vi "CalSet_Control.vi"(8 "error in (no error)":errorcluster, 9 "CalSet Control":enum16{"Save", "Delete", "Load"}(ring), 10 "CalSet Filename (*.cal)":string, 11 "NetA_AgNA in":refnum<class "NetA_AgNA.lvclass">) -> (0 "error out":errorcluster, 3 "NetA_AgNA out":refnum<class "NetA_AgNA.lvclass">)   [LabVIEW 2014, in "NetA_AgNA.lvclass"]
doc: "This allows user to load, save, or delete CalSet files. These files are non-proprietary and stored outside of the Keysight folders."
uses:
  NetA_AgNA.lvclass
  NetA_AgNA.lvclass/NetA_AgNA.ctl
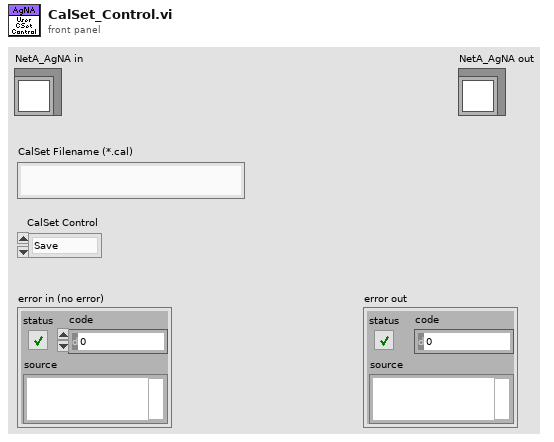
[diagram p1: front panel]
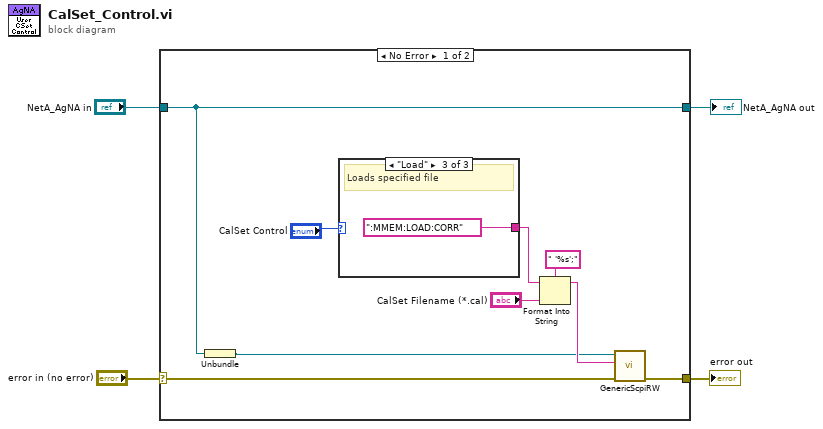
[diagram p0: block diagram]
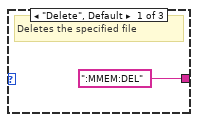
[diagram p2: hidden frame]
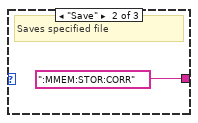
[diagram p3: hidden frame]
diagram:
  n1 = case shown="No Error" "error in (no error)" {
    selector: "error in (no error)" -> [w12 w17]
    tunnel: [w13 w17] -> w4
    tunnel: "NetA_AgNA in" -> [w6 w18]
    tunnel: [w6 w18] -> w1
    frame No Error {
      n2 = Unbundle(w6) -> (w5:refnum<k15>)
      n3 = case shown="\"Load\"" "CalSet Control" {
        tunnel: [":MMEM:DEL" ("Get Dir List") ":MMEM:STOR:CORR" ("Get Dir List") ":MMEM:LOAD:CORR" ("Get Dir List")] -> w11
        frame "Delete", Default {
          # "Deletes the specified file"
        }
        frame "Save" {
          # "Saves specified file"
        }
        frame "Load" {
          # "Loads specified file"
        }
      }
      n4 = Format Into String(format string=" '%s';", initial string=w11, "CalSet Filename (*.cal)") -> (resulting string=w8:string)  [unwired: 1 in, 1 out]
      n5 = call "GenericScpiRW.vi"("error in (no error)"=w12, "SCPI Command"=w8, "resource name"=w5) -> ("error out"=w13:errorcluster)  [unwired: 7 in, 1 out]
    }
    frame Error {
    }
  }
  "error out" <- w4
  "NetA_AgNA out" <- w1
